vi "StringNotifierRef.vi"(11 "String Notifier Refnum":refnum<notifier>) -> (2 "Display string":string, 3 "Stop?":bool)   [LabVIEW 2017]
doc: "Displays the notifier name, the latest notification, the number of VIs or functions currently waiting on the notifier, and the hex value of the reference. You can use this probe to set a breakpoint if the value is an invalid refnum."
uses:
  <vilib>/Utility/error.llb/DialogTypeEnum.ctl
panel:
  in  "error source":string="String Notifier Refnum Probe"
  in  "latest notification":string="Latest notification"
  in  "number waiting":string="Number waiting"
  in  "notifier name":string="Notifier name"
  in  "Pause if Not a Refnum":bool
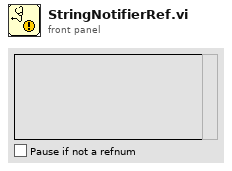
[diagram p1: front panel]
types:
  T1 = typedef "DialogTypeEnum.ctl" = enum16{"no dialog", "OK message", "continue or stop message", "auto error handling dialog", "OK message + warnings", "continue/stop + warnings"}
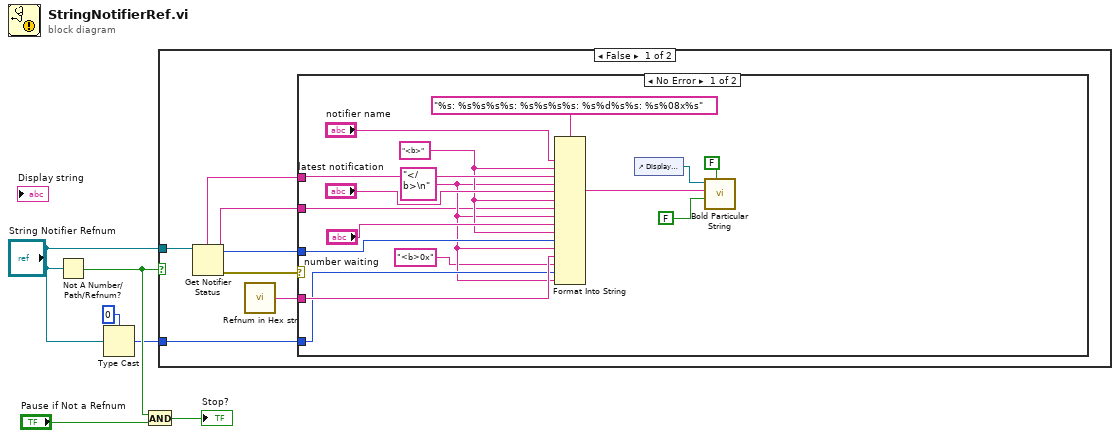
[diagram p0: block diagram]
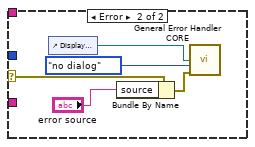
[diagram p2: hidden frame]
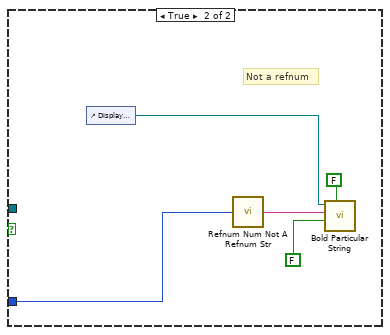
[diagram p3: hidden frame]
diagram:
  n1 = Not A Number/Path/Refnum?(number/path/refnum="String Notifier Refnum") -> (NaN/Path/Refnum?=w4:bool)
  n2 = Type Cast(type=u32 0, x="String Notifier Refnum") -> (*(type *) &x=w1:u32)
  n3 = And(x=w4, y="Pause if Not a Refnum") -> (x .and. y?=→"Stop?":bool)
  n4 = case shown="False" w4 {
    tunnel: "String Notifier Refnum" -> [w13 _]
    tunnel: w1 -> [w7 w36]
    frame False {
      n5 = Get Notifier Status(notifier=w13) -> (notifier name=w12:string, current notification=w10:string, # waiting=w11:i32, error out=w9:errorcluster)  [unwired: 1 in, 1 out]
      n6 = call <vilib>:"Refnum in Hex str.vi"() -> ("refnum in hex"=w8:string)
      n7 = case shown="No Error" w9 {
        selector: w9 -> [_ w32]
        tunnel: w7 -> [w18 _]
        tunnel: w12 -> [w24 _]
        tunnel: w11 -> [w21 _]
        tunnel: w8 -> [w20 _]
        tunnel: w10 -> [w15 _]
        frame No Error {
          w17 = "</b>\n"
          w19 = "<b>"
          n8 = Format Into String(format string="%s: %s%s%s%s: %s%s%s%s: %s%d%s%s: %s%08x%s", "notifier name", w19, w24, w17, "latest notification", w19, w15, w17, "number waiting", w19, w21, w17, w20, "<b>0x", w18, w17) -> (resulting string=w28:string)  [unwired: 2 in, 1 out]
          n9 = control-ref of="Display string"() -> (w29:refnum<vi>)
          n10 = call <vilib>:"Bold Particular String.vi"("Always Refresh? (TRUE)"=FALSE ("Always Refresh? (FALSE)"), "resize string? (TRUE)"=FALSE ("resize string?"), "text to display"=w28, "string refnum"=w29) -> ()  [unwired: 6 in, 2 out]
        }
        frame Error {
          n11 = control-ref of="Display string"() -> (w31:refnum<vi>)
          n12 = Bundle By Name(cluster=w32, "source"="error source") -> (w33:errorcluster)
          n13 = call <vilib>:"General Error Handler CORE.vi"("String to Format (not a refnum)"=w31, "type of dialog (OK msg:1)"=DialogTypeEnum."no dialog", "error in (no error)"=w33) -> ()  [unwired: 7 in, 6 out]
        }
      }
    }
    frame True {
      # "Not a refnum"
      n14 = control-ref of="Display string"() -> (w38:refnum<vi>)
      n15 = call <vilib>:"Refnum Num Not A Refnum Str.vi"("Numeric"=w36) -> ("text to display"=w35:string)
      n16 = call <vilib>:"Bold Particular String.vi"("Always Refresh? (TRUE)"=FALSE ("Always Refresh? (FALSE)"), "resize string? (TRUE)"=FALSE, "text to display"=w35, "string refnum"=w38) -> ()  [unwired: 6 in, 2 out]
    }
  }
